vi "Add Topic Subscriber.vi"(8 "error in (no error)":errorcluster, 10 "SubscriptionRequest":refnum<class "SubscriptionRequest.lvclass">, 11 "Topic in":refnum<class "Topic.lvclass">) -> (0 "error out":errorcluster, 3 "Topic out":refnum<class "Topic.lvclass">)   [LabVIEW 2015, in "Mediator.lvlib" / "Topic.lvclass"]
doc: "<License>\nCopyright © 2017 Composed Systems, LLC | All rights reserved\nwww.composed.io\n\nAuthor: Ethan Stern <ethan.stern@composed.io>\n\nThis software is provided \"AS IS\" WITHOUT WARRANTIES, either express or implied, AND IS FOR EDUCATIONAL PURPOSES ONLY.\n</License>"
uses:
  Topic.lvclass
  IMediator/SubscriptionRequest/SubscriptionRequest.lvclass
  Topic.lvclass/Topic.ctl
  IMediator/ISubscriptionPolicy/ISubscriptionPolicy.lvclass
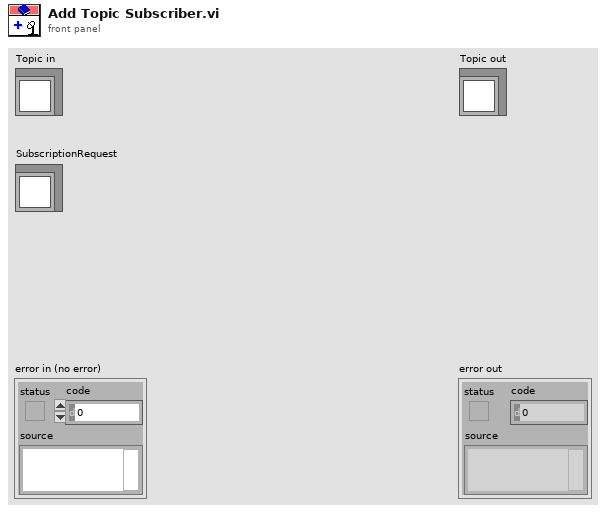
[diagram p1: front panel]
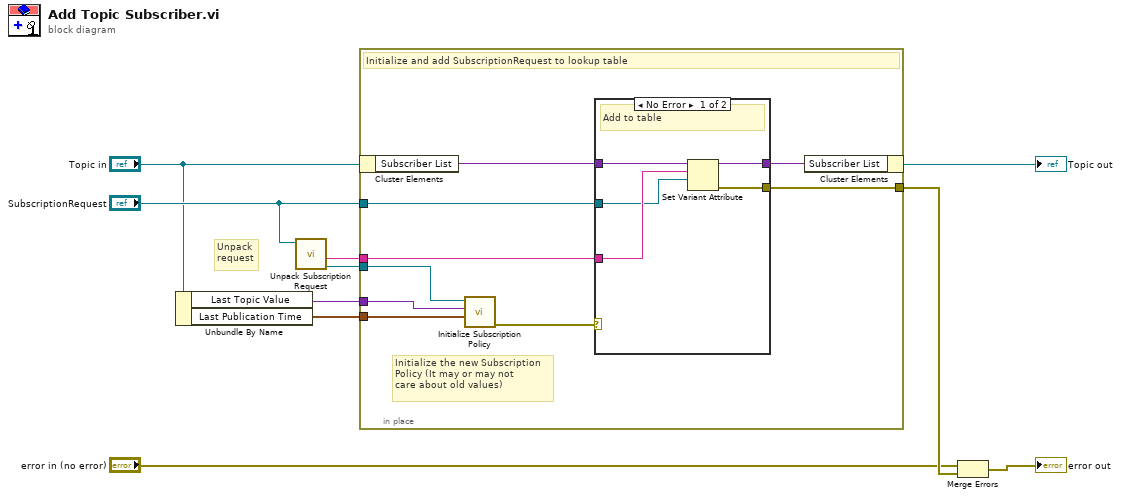
[diagram p0: block diagram]
diagram:
  # "Unpack\nrequest"
  n1 = Unbundle By Name("Topic in") -> ("Last Topic Value"=w2:variant, "Last Publication Time"=w1:timestamp)
  n2 = call "Unpack Subscription Request.vi"("SubscriptionRequest in"="SubscriptionRequest") -> ("Subscription Policy"=w4:refnum<data-value>, "Unique Subscriber ID"=w6:string)  [unwired: 7 in, 2 out]
  n3 = in-place {
    in-place-border: [w17] -> w10
    in-place-border: w6 -> [w16]
    in-place-border: "SubscriptionRequest" -> [w15]
    in-place-border: w4 -> [w14]
    in-place-border: w2 -> [w13]
    in-place-border: w1 -> [w11]
    # "Initialize the new Subscription\nPolicy (It may or may not\ncare about old values)"
    # "Initialize and add SubscriptionRequest to lookup table"
    n4 = in-place-cluster #1("Topic in") -> ("Subscriber List"=w19:variant)
    n5 = call "Initialize Subscription Policy.vi"("Last Publish Time"=w11, "Last Topic Value"=w13, "Subscription Policy"=w14) -> ("error out"=w12:errorcluster)  [unwired: 8 in]
    n6 = case shown="No Error" w12 {
      tunnel: w19 -> [w24 w25]
      tunnel: [w23 w25] -> w18
      tunnel: [w22 _] -> w17
      tunnel: w16 -> [w21 _]
      tunnel: w15 -> [w20 _]
      frame No Error {
        # "Add to table"
        n7 = Set Variant Attribute(Variant=w24, name=w21, value=w20) -> (Variant out=w23:variant, error out=w22:errorcluster)  [unwired: 1 in, 1 out]
      }
      frame Error {
        # "Policy is not valid --\nDo not add to table"
        # "A rough start"
      }
    }
    n8 = in-place-cluster #1("Subscriber List"=w18) -> (→"Topic out":refnum<class "Topic.lvclass">)
  }
  n9 = Merge Errors("error in (no error)", w10) -> (→"error out":errorcluster)
